vi "Print VI.vi"(6 "Images Destination":path, 8 "Error In":errorcluster, 11 "VI In":refnum<vi>) -> (0 "Error Out":errorcluster, 3 "VI Out":refnum<vi>)   [LabVIEW 2018, in "Scripts.lvlib"]
uses:
  Scripts.lvlib
  <vilib>/Field R&D Services/Labricator/Toolkit/Labricator.lvlib
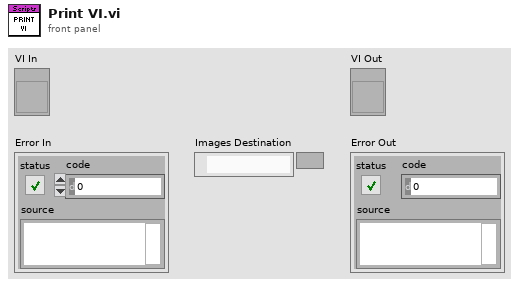
[diagram p1: front panel]
types:
  T1 = enum32{"Custom", "Standard", "Using Panel", "Using SubVI", "Complete"}
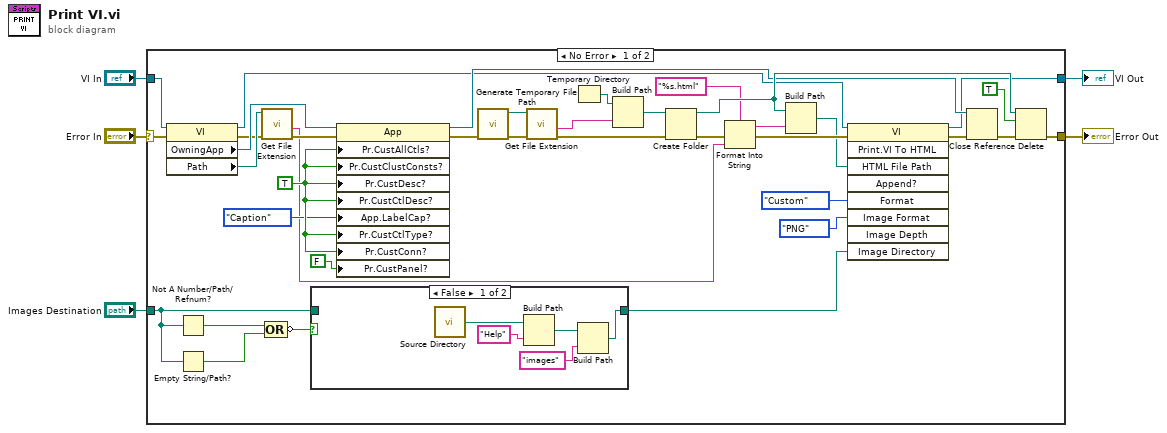
[diagram p0: block diagram]
diagram:
  n1 = case shown="No Error" "Error In" {
    selector: "Error In" -> [w15 w49]
    tunnel: [w41 w49] -> w5
    tunnel: [w19 w50] -> w4
    tunnel: "VI In" -> [w18 w50]
    tunnel: "Images Destination" -> [w7 _]
    frame No Error {
      w25 = TRUE ("Printing:Custom All Controls?")
      n2 = property class="VI"(reference=w18, error in=w15) -> (reference out=w17:refnum<vi>, error out=w13:errorcluster, "OwningApp"=w16:refnum<vi>, "Path"=w14:path)
      n3 = Not A Number/Path/Refnum?(number/path/refnum=w7) -> (NaN/Path/Refnum?=w9:bool)
      n4 = Empty String/Path?(string/path=w7) -> (empty?=w10:bool)
      n5 = call <vilib>:"Get File Extension.vi"("error in (no error)"=w13, "file"=w14) -> ("error out"=w12:errorcluster, "filename without extension"=w11:string)  [unwired: 5 in, 3 out]
      n6 = Compound Arithmetic op=OR(w9, w10) -> (invert w8:bool)
      n7 = case shown="False" w8 {
        tunnel: w7 -> [_ w48]
        tunnel: [w43 w48] -> w6
        frame False {
          n8 = call <vilib>:"Source Directory.vi"() -> ("Source Directory"=w47:path)
          n9 = Build Path(base path=w47, name or relative path="Help") -> (appended path=w45:path)
          n10 = Build Path(base path=w45, name or relative path="images") -> (appended path=w43:path)
        }
        frame True {
        }
      }
      n11 = property class="App"(reference=w16, error in=w12, "Pr.CustAllCtls?"=w25, "Pr.CustClustConsts?"=w25, "Pr.CustDesc?"=w25, "Pr.CustCtlDesc?"=w25, "App.LabelCap?"=enum16{"Label", "Caption", "Caption[Label]"}."Caption" ("Printing:Custom Control Label/Caption?"), "Pr.CustCtlType?"=w25, "Pr.CustConn?"=w25, "Pr.CustPanel?"=FALSE ("Printing:Custom Panel?")) -> (reference out=w23:refnum<vi>, error out=w27:errorcluster)
      n12 = call <vilib>:"Generate Temporary File Path.vi"("error in (no error)"=w27) -> ("error out"=w38:errorcluster, "Unique Temporary File Path"=w33:path)  [unwired: 9 in]
      n13 = call <vilib>:"Get File Extension.vi"("error in (no error)"=w38, "file"=w33) -> ("error out"=w37:errorcluster, "filename without extension"=w35:string)  [unwired: 5 in, 3 out]
      n14 = Temporary Directory() -> (w34:path)
      n15 = Build Path(base path=w34, name or relative path=w35) -> (appended path=w36:path)
      n16 = Create Folder(path (use dialog)=w36, error in=w37) -> (created path=w39:path, error out=w28:errorcluster)  [unwired: 1 in, 1 out]
      n17 = Format Into String(format string="%s.html", error in=w28, w11) -> (resulting string=w32:string, error out=w30:errorcluster)  [unwired: 1 in]
      n18 = Build Path(base path=w39, name or relative path=w32) -> (appended path=w29:path)
      n19 = invoke class="VI" method="Print.VI To HTML"(reference=w17, error in=w30, "HTML File Path"=w29, "Format"=T1."Custom", "Image Format"=enum32{"PNG", "JPEG", "GIF"}."PNG", "Image Directory"=w6) -> (reference out=w19:refnum<vi>, error out=w20:errorcluster)  [unwired: 3 in, 7 out]
      n20 = Close Reference(reference=w23, error in (no error)=w20) -> (error out=w40:errorcluster)
      n21 = Delete(path (use dialog)=w39, entire hierarchy (F)=TRUE, error in=w40) -> (error out=w41:errorcluster)  [unwired: 2 in, 2 out]
    }
    frame Error {
    }
  }
  "Error Out" <- w5
  "VI Out" <- w4
